vi "Run CLI Action.vi"(8 "error in (no error)":errorcluster, 11 "CLI in":refnum<class "CLI.lvclass">) -> (0 "error out":errorcluster)   [LabVIEW 2020, in "neg-pkg-cli.lvlib" / "CLI.lvclass"]
uses:
  CLI.lvclass
  CLI.lvclass/CLI.ctl
  build/ppl/neg-pkg.lvlibp/Action/Action.lvclass
  MGI Console/Source/Console/Console.lvclass
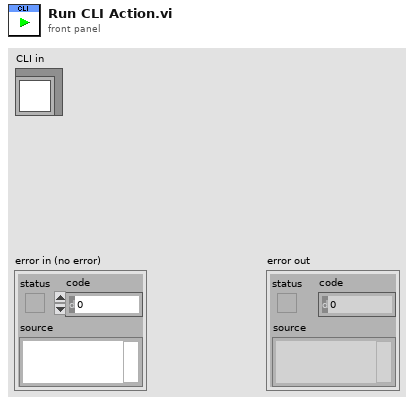
[diagram p1: front panel]
types:
  T1 = typedef "neg-pkg.lvlibp/Action.lvclass/Run Parameters.ctl" = cluster{"Status":refnum<class "Status.lvclass">, "Working Directory":path}
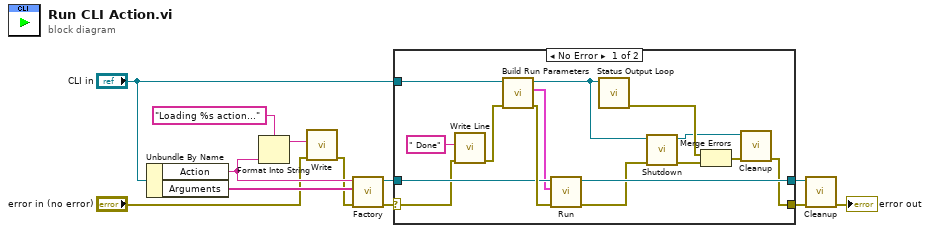
[diagram p0: block diagram]
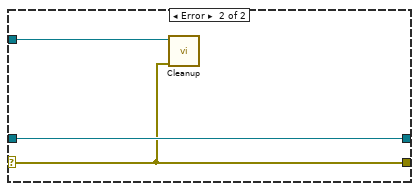
[diagram p2: hidden frame]
diagram:
  n1 = Unbundle By Name("CLI in") -> ("Action"=w4:string, "Arguments"=w7:string[])
  n2 = Format Into String(format string="Loading %s action...", w4) -> (resulting string=w2:string)  [unwired: 2 in, 1 out]
  n3 = call "Write.vi"("error in (no error)"="error in (no error)", "String"=w2) -> ("error out"=w1:errorcluster)  [unwired: 9 in]
  n4 = call "Factory.vi"("error in (no error)"=w1, "Args"=w7, "Action Name"=w4) -> ("error out"=w12:errorcluster, "Action"=w11:refnum<class "Action.lvclass">)  [unwired: 7 in]
  n5 = case shown="No Error" w12 {
    selector: w12 -> [w18 w28]
    tunnel: w11 -> [w26 w30]
    tunnel: [w25 w30] -> w10
    tunnel: [w14 w28] -> w9
    tunnel: "CLI in" -> [w24 w29]
    frame No Error {
      n6 = call "Write Line.vi"("error in (no error)"=w18, "Line"=" Done") -> ("error out"=w17:errorcluster)  [unwired: 9 in]
      n7 = call "Build Run Parameters.vi"("error in (no error)"=w17, "CLI in"=w24) -> ("error out"=w27:errorcluster, "Run Parameters"=w23:T1, "CLI out"=w21:refnum<class "CLI.lvclass">)  [unwired: 7 in]
      n8 = call "Run.vi"("error in (no error)"=w27, "Run Parameters"=w23, "Action in"=w26) -> ("error out"=w22:errorcluster, "Action out"=w25:refnum<class "Action.lvclass">)  [unwired: 7 in]
      n9 = call "Status Output Loop.vi"("CLI in"=w21) -> ("error out"=w19:errorcluster)  [unwired: 9 in, 1 out]
      n10 = call "Shutdown.vi"("error in (no error)"=w22, "CLI in"=w21) -> ("error out"=w20:errorcluster, "CLI out"=w13:refnum<class "CLI.lvclass">)  [unwired: 8 in]
      n11 = Merge Errors(w19, w20) -> (w15:errorcluster)
      n12 = call "Cleanup.vi"("error in (no error)"=w15, "CLI in"=w13) -> ("error out"=w14:errorcluster)  [unwired: 9 in]
    }
    frame Error {
      n13 = call "Cleanup.vi"("error in (no error)"=w28, "CLI in"=w29) -> ()  [unwired: 9 in, 1 out]
    }
  }
  n14 = call "Cleanup.vi"("error in (no error)"=w9, "Action in"=w10) -> ("error out"=→"error out":errorcluster)  [unwired: 8 in, 1 out]
